vi "NTCP Network Parameters DAO.vi"(7 "refnum":T2, 8 "error in (no error)":errorcluster, 10 "Network Parameters In":T1={"Port Number"=0, "Notification Name"="DataAvailableForTransmission", "Wait For Notification Timeout"=1000}, 11 "Persistent DAO Actions":T3) -> (0 "error out":errorcluster, 3 "Network Parameters Out":T1={"Port Number"=0, "Notification Name"="DataAvailableForTransmission", "Wait For Notification Timeout"=1000}, 4 "refnum out":T2)   [LabVIEW 2009]
uses:
  Network Parameters.ctl
  Metadata/Persistant DAO Actions.ctl
  <vilib>/Utility/config.llb/Config Data RefNum.ctl
  <vilib>/Utility/config.llb/NI_LVConfig.lvlib
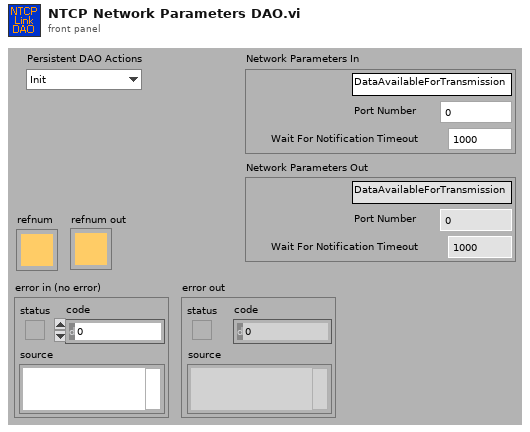
[diagram p1: front panel]
types:
  T1 = typedef "Network Parameters.ctl" = cluster{"Port Number":u16, "Notification Name":string, "Wait For Notification Timeout":i32}
  T2 = typedef "NI_LVConfig.lvlib/Config Data RefNum.ctl" = refnum<k1>
  T3 = typedef "Persistant DAO Actions.ctl" = enum16{"Init", "Get", "Set", "Load", "Save"}
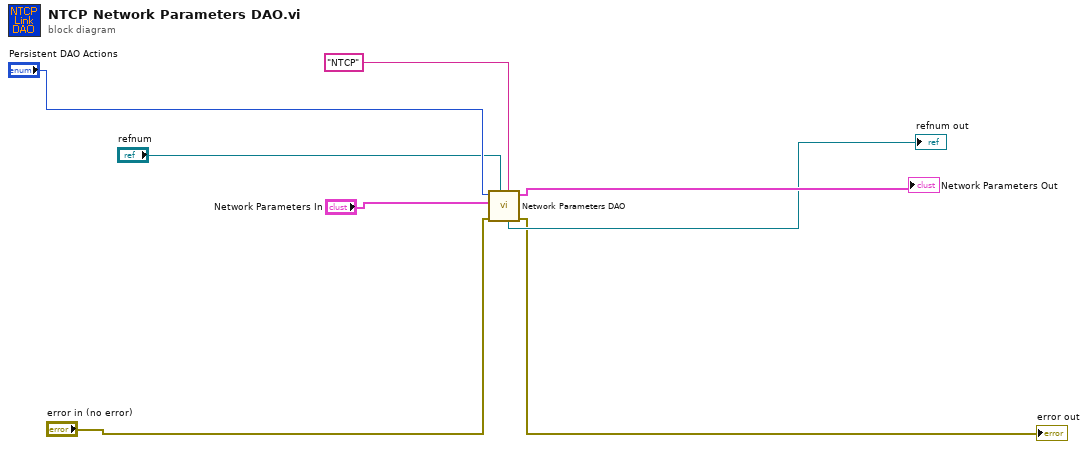
[diagram p0: block diagram]
diagram:
  n1 = call "Network Parameters DAO.vi"("Section"="NTCP", "refnum"="refnum", "error in (no error)"="error in (no error)", "Network Parameters In"="Network Parameters In", "Persistent DAO Actions"="Persistent DAO Actions") -> ("error out"=→"error out":errorcluster, "Network Parameters Out"=→"Network Parameters Out":T1, "refnum out"=→"refnum out":T2)  [unwired: 4 in]
